vi "Shut Down.vi"(8 "error in":errorcluster, 11 "LTB-1 in":refnum<class "LTB-1.lvclass">) -> (0 "error out":errorcluster, 3 "LTB-1 out":refnum<class "LTB-1.lvclass">)   [LabVIEW 2017, in "LTB-1.lvlib" / "LTB-1.lvclass"]
doc: "This is a dynamically dispatched VI, the parent method assures that the shutter is closed, the child routine will determine all of the additional steps required to effectively shut down the EXFO unit\n\nAuthor: Ron Dexter\nCompany: Luminar\nModified: 5/20/2018"
uses:
  LTB-1.lvclass
  APD Sensitivity Calibration/VIs/Instruments/EXFO/EXFO.lvlibp/EXFO.lvclass
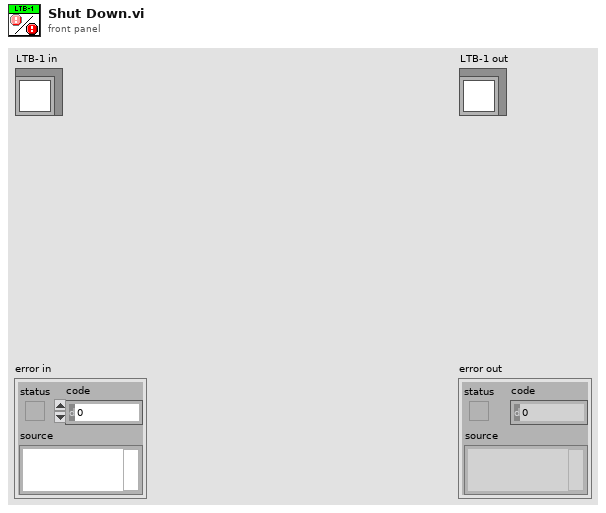
[diagram p1: front panel]
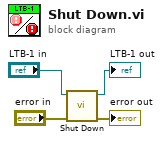
[diagram p0: block diagram]
diagram:
  n1 = call-parent "Shut Down.vi"("error in"="error in", "EXFO in"="LTB-1 in") -> ("error out"=→"error out":errorcluster, "EXFO out"=→"LTB-1 out":refnum<class "LTB-1.lvclass">)  [unwired: 8 in]
